vi "Blade Coater Low Level Write.vi"(7 "Solution ID":i32, 8 "error in (no error)":errorcluster, 9 "Current Layer ID":i32, 10 "Layer Information Cluster":T2 {"Deposition Method" items=["Blade Coating", "Spin Coating", "Thermal Evaporation", "E-Beam Evaporation", "Sputtering", "Drop Casting", "Dip Coating", "Pulsed Laser Deposition", "Chemival Vapour Deposition", "Atomic Layer Deposition", "Spray Coating", "Screen Printing", "Electroplating", "Molecular Beam Epitaxy", "Custom Deposition"]; "Layer Type" items=["Front Electrode", "Electron Transport Layer", "Active Layer", "Hole Transport Layer", "Back Electrode", "Custom Layer"]}, 11 "Refnum in":T1) -> (0 "error out":errorcluster, 3 "Refnum out":T1)   [LabVIEW 2020]
uses:
  Data Clusters/Layer Information Cluster.ctl
  <vilib>/addons/database/Connection.llb/Conn ObjectReference.ctl
  <vilib>/addons/database/NI_Database_API.lvlib
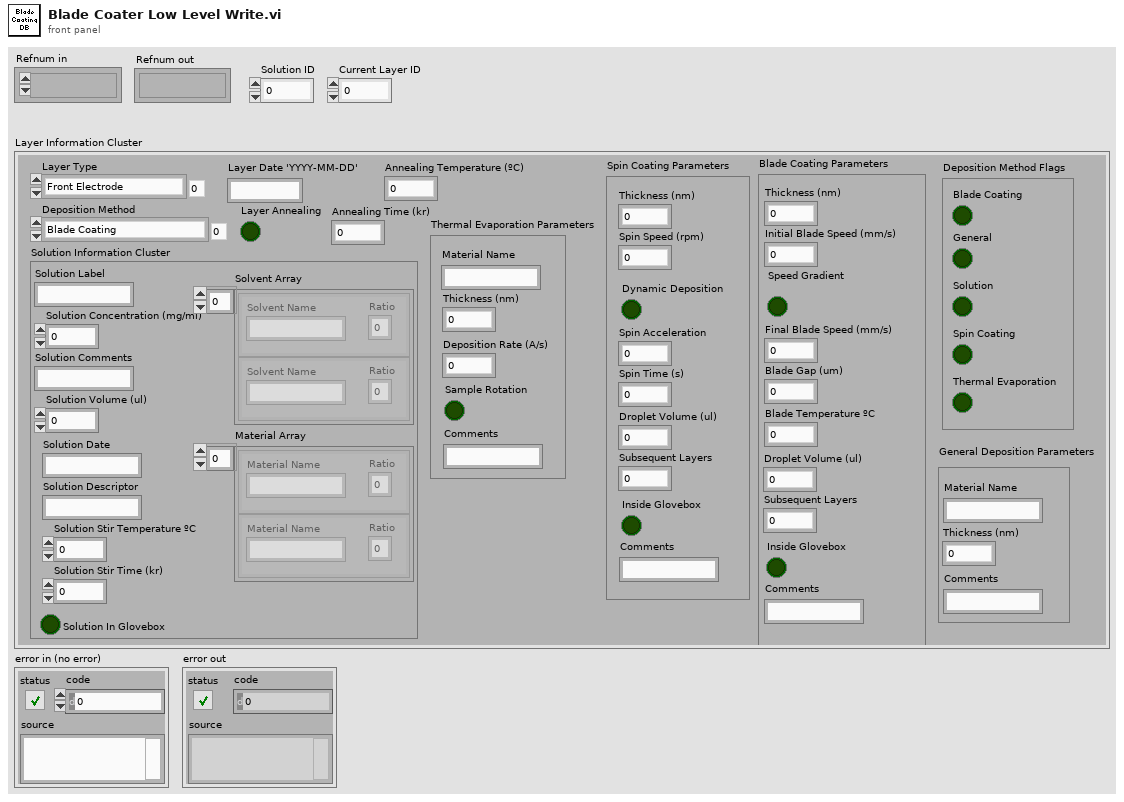
[diagram p1: front panel]
types:
  T1 = typedef "NI_Database_API.lvlib/Conn ObjectReference.ctl" = refnum<k1>
  T2 = typedef "Layer Information Cluster.ctl" = cluster{"Solution Information Cluster":cluster{"Solution Label":string, "Solution Concentration (mg/ml)":dbl, "Solution Comments ":string, "Solution Volume (ul) ":dbl, "Solution Date ":string, "Solution Descriptor ":string, "Solution Stir Temperature ºC ":dbl, "Solution Stir Time (kr) ":dbl, "Solution In Glovebox":bool, "Solvent Array":cluster{"Solvent Name":string, "Ratio":dbl}[], "Material Array":cluster{"Material Name":string, "Ratio":dbl}[]}, "Layer Type":u16, "Deposition Method":u16, "Layer Annealing":bool, "General Deposition Parameters":cluster{"Thickness (nm)":dbl, "Comments":string, "Material Name":string}, "Blade Coating Parameters":cluster{"Thickness (nm)":dbl, "Initial Blade Speed (mm/s)":dbl, "Speed Gradient":bool, "Final Blade Speed (mm/s)":dbl, "Blade Gap (um)":dbl, "Droplet Volume (ul)":dbl, "Subsequent Layers":dbl, "Inside Glovebox":bool, "Comments":string, "Blade Temperature ºC":dbl}, "Spin Coating Parameters":cluster{"Thickness (nm)":dbl, "Spin Speed (rpm)":dbl, "Dynamic Deposition":bool, "Spin Acceleration":dbl, "Spin Time (s)":dbl, "Droplet Volume (ul)":dbl, "Subsequent Layers":dbl, "Inside Glovebox":bool, "Comments":string}, "Thermal Evaporation Parameters":cluster{"Deposition Rate (A/s)":dbl, "Thickness (nm)":dbl, "Comments":string, "Material Name":string, "Sample Rotation":bool}, "Layer Date 'YYYY-MM-DD'":string, "Annealing Time (kr)":dbl, "Annealing Temperature (ºC)":dbl, "Deposition Method Flags":cluster{"Blade Coating":bool, "General ":bool, "Solution":bool, "Spin Coating":bool, "Thermal Evaporation":bool}}
  T3 = cluster{"Thickness (nm)":dbl, "Spin Speed (rpm)":dbl, "Dynamic Deposition":bool, "Spin Acceleration":dbl, "Spin Time (s)":dbl, "Droplet Volume (ul)":dbl, "Subsequent Layers":dbl, "Inside Glovebox":bool, "Comments":string, "Current Layer ID":i32}
  T4 = cluster{"Solution ID":i32, "Thickness (nm)":dbl, "Initial Blade Speed (mm/s)":dbl, "Final Blade Speed (mm/s)":dbl, "Speed Gradient":bool, "Blade Gap (um)":dbl, "Blade Temperature ºC":dbl, "Droplet Volume (ul)":dbl, "Subsequent Layers":dbl, "Inside Glovebox":bool, "Comments":string, "Current Layer ID":i32}
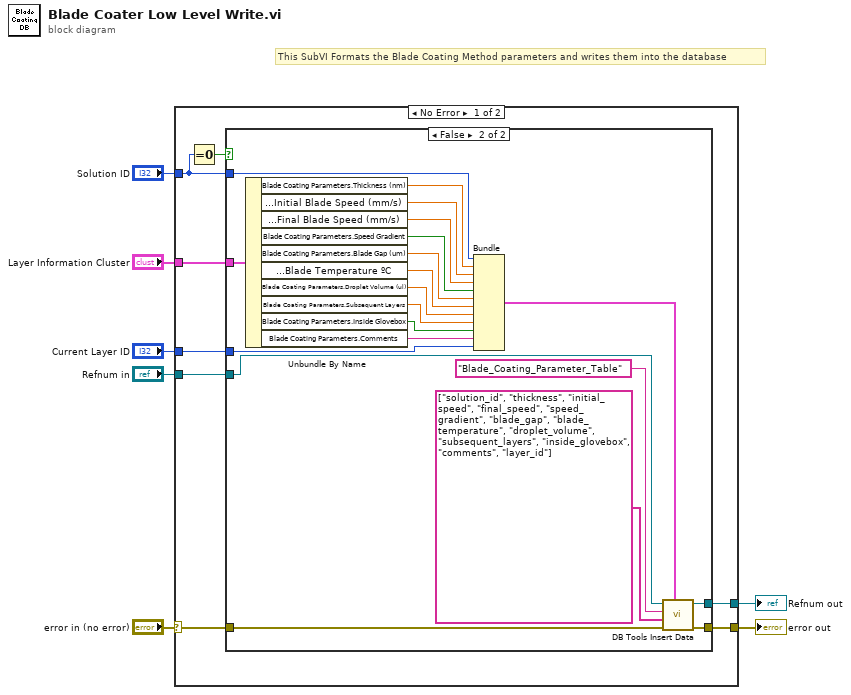
[diagram p0: block diagram]
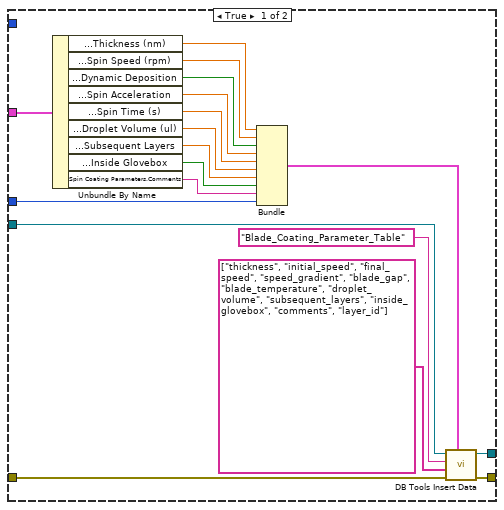
[diagram p2: hidden frame]
diagram:
  # "This SubVI Formats the Blade Coating Method parameters and writes them into the database"
  n1 = case shown="No Error" "error in (no error)" {
    selector: "error in (no error)" -> [w12 w54]
    tunnel: "Solution ID" -> [w15 _]
    tunnel: "Current Layer ID" -> [w13 _]
    tunnel: "Refnum in" -> [w11 w55]
    tunnel: [w10 w55] -> w3
    tunnel: [w9 w54] -> w2
    tunnel: "Layer Information Cluster" -> [w8 _]
    frame No Error {
      n2 = Equal To 0?(x=w15) -> (x = 0?=w14:bool)
      n3 = case shown="False" w14 {
        tunnel: [w33 w53] -> w9
        tunnel: [w32 w52] -> w10
        tunnel: w11 -> [w31 w51]
        tunnel: w12 -> [w30 w50]
        tunnel: w13 -> [w18 w47]
        tunnel: w8 -> [w29 w49]
        tunnel: w15 -> [_ w44]
        frame True {
          n4 = Unbundle By Name(w29) -> ("Spin Coating Parameters.Thickness (nm)"=w27:dbl, "Spin Coating Parameters.Spin Speed (rpm)"=w26:dbl, "Spin Coating Parameters.Dynamic Deposition"=w25:bool, "Spin Coating Parameters.Spin Acceleration"=w24:dbl, "Spin Coating Parameters.Spin Time (s)"=w23:dbl, "Spin Coating Parameters.Droplet Volume (ul)"=w22:dbl, "Spin Coating Parameters.Subsequent Layers"=w21:dbl, "Spin Coating Parameters.Inside Glovebox"=w20:bool, "Spin Coating Parameters.Comments"=w19:string)
          n5 = Bundle("Thickness (nm)"=w27, "Spin Speed (rpm)"=w26, "Dynamic Deposition"=w25, "Spin Acceleration"=w24, "Spin Time (s)"=w23, "Droplet Volume (ul)"=w22, "Subsequent Layers"=w21, "Inside Glovebox"=w20, "Comments"=w19, "Current Layer ID"=w18) -> (w17:T3)  [unwired: 1 in]
          n6 = call <vilib>:"DB Tools Insert Data.vi"("data"=w17, "error in (no error)"=w30, "columns"=string[] ["thickness", "initial_speed", "final_speed", "speed_gradient", "blade_gap", "blade_temperature", "droplet_volume", "subsequent_layers", "inside_glovebox", "comments", "layer_id"], "table"="Blade_Coating_Parameter_Table", "connection reference"=w31) -> ("error out"=w33:errorcluster, "connection reference out"=w32:T1)  [unwired: 5 in]
        }
        frame False {
          n7 = Unbundle By Name(w49) -> ("Blade Coating Parameters.Thickness (nm)"=w43:dbl, "Blade Coating Parameters.Initial Blade Speed (mm/s)"=w42:dbl, "Blade Coating Parameters.Final Blade Speed (mm/s)"=w41:dbl, "Blade Coating Parameters.Speed Gradient"=w40:bool, "Blade Coating Parameters.Blade Gap (um)"=w39:dbl, "Blade Coating Parameters.Blade Temperature ºC"=w38:dbl, "Blade Coating Parameters.Droplet Volume (ul)"=w37:dbl, "Blade Coating Parameters.Subsequent Layers"=w36:dbl, "Blade Coating Parameters.Inside Glovebox"=w35:bool, "Blade Coating Parameters.Comments"=w34:string)
          n8 = Bundle("Solution ID"=w44, "Thickness (nm)"=w43, "Initial Blade Speed (mm/s)"=w42, "Final Blade Speed (mm/s)"=w41, "Speed Gradient"=w40, "Blade Gap (um)"=w39, "Blade Temperature ºC"=w38, "Droplet Volume (ul)"=w37, "Subsequent Layers"=w36, "Inside Glovebox"=w35, "Comments"=w34, "Current Layer ID"=w47) -> (w46:T4)  [unwired: 1 in]
          n9 = call <vilib>:"DB Tools Insert Data.vi"("data"=w46, "error in (no error)"=w50, "columns"=string[] ["solution_id", "thickness", "initial_speed", "final_speed", "speed_gradient", "blade_gap", "blade_temperature", "droplet_volume", "subsequent_layers", "inside_glovebox", "comments", "layer_id"], "table"="Blade_Coating_Parameter_Table", "connection reference"=w51) -> ("error out"=w53:errorcluster, "connection reference out"=w52:T1)  [unwired: 5 in]
        }
      }
    }
    frame Error {
    }
  }
  "Refnum out" <- w3
  "error out" <- w2
